vi "Inflation Results to String.vi"(10 "comments":string, 11 "results":T1) -> (3 "Results String":string)   [LabVIEW 2020]
uses:
  Controller Loop/Controller Data.ctl
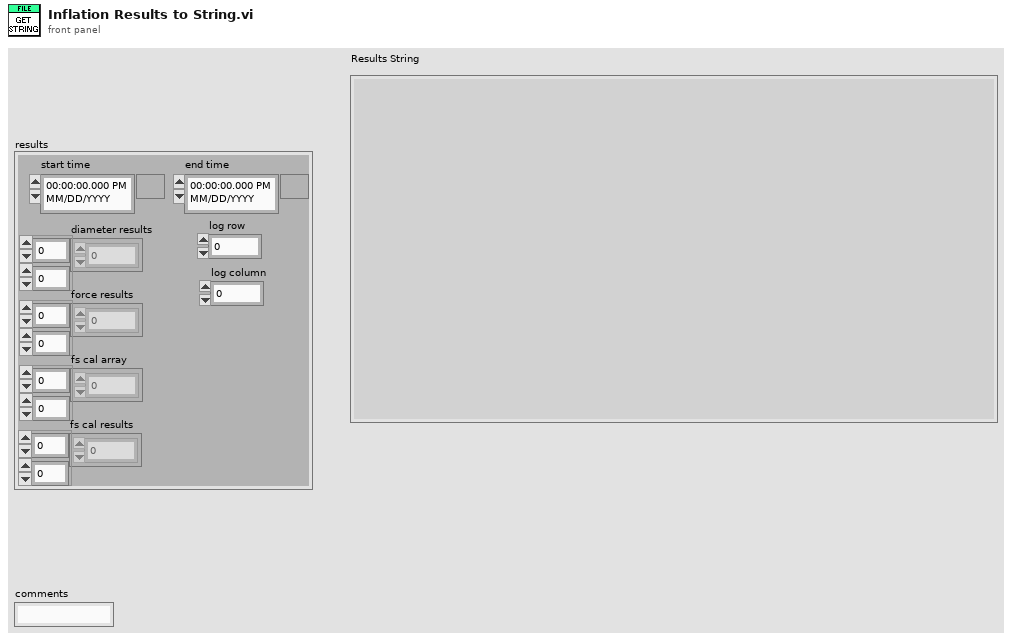
[diagram p1: front panel]
types:
  T1 = typedef "Controller Data.ctl" = cluster{"diameter results":dbl[][], "force results":dbl[][], "fs cal array":dbl[][], "fs cal results":dbl[][], "start time":timestamp, "end time":timestamp, "log row":i32, "log column":i32}
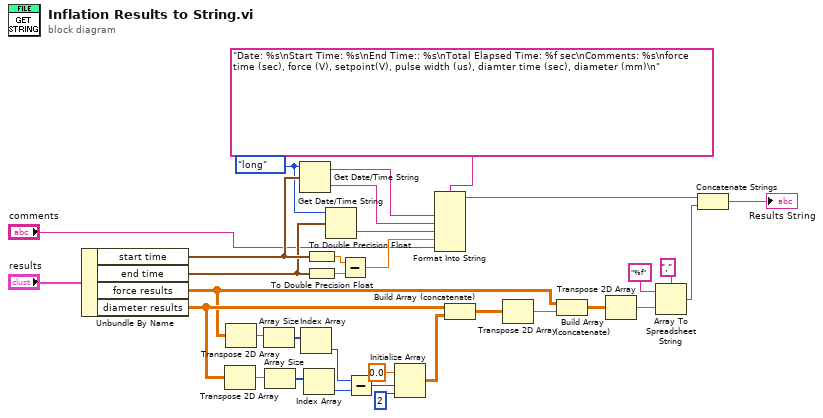
[diagram p0: block diagram]
diagram:
  w22 = enum16{"short", "long", "abbreviated"}."long" ("date format (0)")
  n1 = Unbundle By Name("results") -> ("start time"=w23:timestamp, "end time"=w21:timestamp, "force results"=w3:dbl[][], "diameter results"=w5:dbl[][])
  n2 = Transpose 2D Array(2D array=w5) -> (transposed array=w4:dbl[][])
  n3 = Transpose 2D Array(2D array=w3) -> (transposed array=w6:dbl[][])
  n4 = Array Size(array=w6) -> (size(s)=w20:i32[])
  n5 = Array Size(array=w4) -> (size(s)=w19:i32[])
  n6 = Get Date/Time String(date format (0)=w22, seconds (now)=w23) -> (date string=w29:string, time string=w28:string)  [unwired: 1 in]
  n7 = Index Array(array=w20) -> (element=w18:i32)  [unwired: 1 in]
  n8 = Index Array(array=w19) -> (element=w17:i32)  [unwired: 1 in]
  n9 = To Double Precision Float(number=w23) -> (double precision float=w31:dbl)
  n10 = To Double Precision Float(number=w21) -> (double precision float=w32:dbl)
  n11 = Get Date/Time String(date format (0)=w22, seconds (now)=w21) -> (time string=w27:string)  [unwired: 1 in, 1 out]
  n12 = Subtract(x=w31, y=w32) -> (x-y=w30:dbl)
  n13 = Subtract(x=w18, y=w17) -> (x-y=w16:i32)
  n14 = Initialize Array(0.0 ("element"), w16, 2 ("dimension size")) -> (w13:dbl[][])
  n15 = Format Into String(format string="Date: %s\nStart Time: %s\nEnd Time:: %s\nTotal Elapsed Time: %f sec\nComments: %s\nforce time (sec), force (V), setpoint(V), pulse width (us), diamter time (sec), diameter (mm)\n", w29, w28, w27, w30, "comments") -> (resulting string=w26:string)  [unwired: 2 in, 1 out]
  n16 = Build Array (concatenate)(w5, w13) -> (w2:dbl[][])
  n17 = Transpose 2D Array(2D array=w2) -> (transposed array=w1:dbl[][])
  n18 = Build Array (concatenate)(w3, w1) -> (w9:dbl[][])
  n19 = Transpose 2D Array(2D array=w9) -> (transposed array=w8:dbl[][])
  n20 = Array To Spreadsheet String(delimiter (Tab)=",", array=w8, 3:"%f" ("format string")) -> (spreadsheet string=w10:string)
  n21 = Concatenate Strings(w26, w10) -> (→"Results String":string)
